vi "fruitWay.vi"() -> ()   [LabVIEW 2014]
uses:
  <vilib>/Utility/file.llb/Write To Spreadsheet File (DBL).vi
panel:
  out "appended array":dbl[][](array[numeric])
  out "Array 2":dbl[](array[numeric])
  out "Array":dbl[](array[numeric])
  in  "Boolean":bool
  in  "initial angle":dbl
  in  "initial velocity":dbl
  in  "Position:Top":i32
  in  "Position:Left":i32
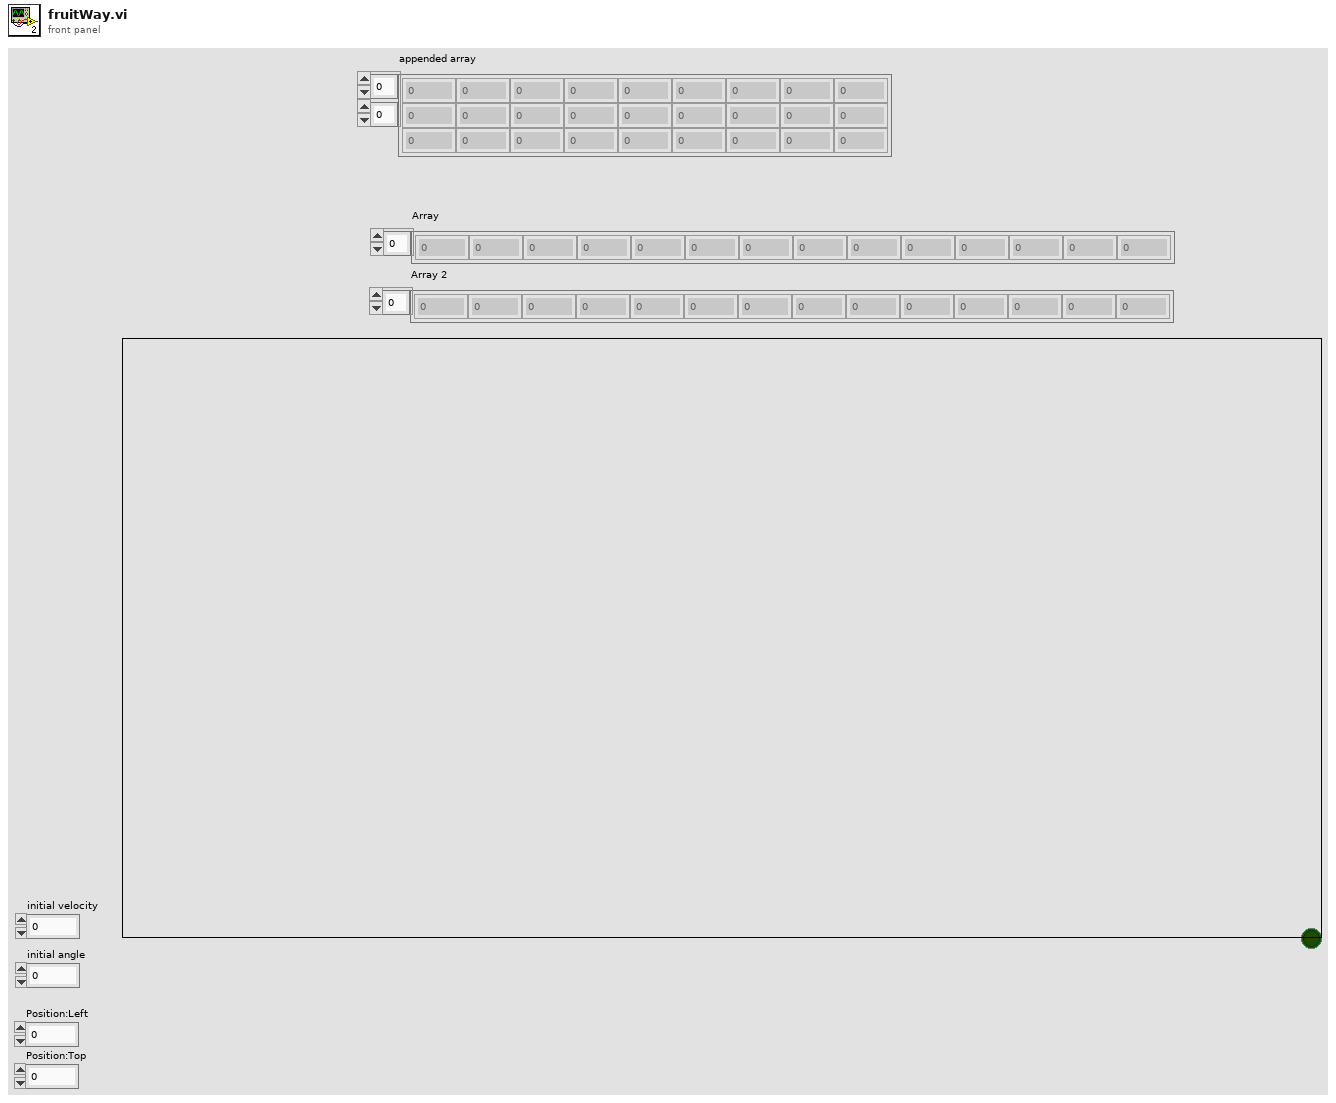
[diagram p1: front panel]
types:
  T1 = typedef "LVPositionTypeDef.ctl" = cluster{"Left":i32, "Top":i32}
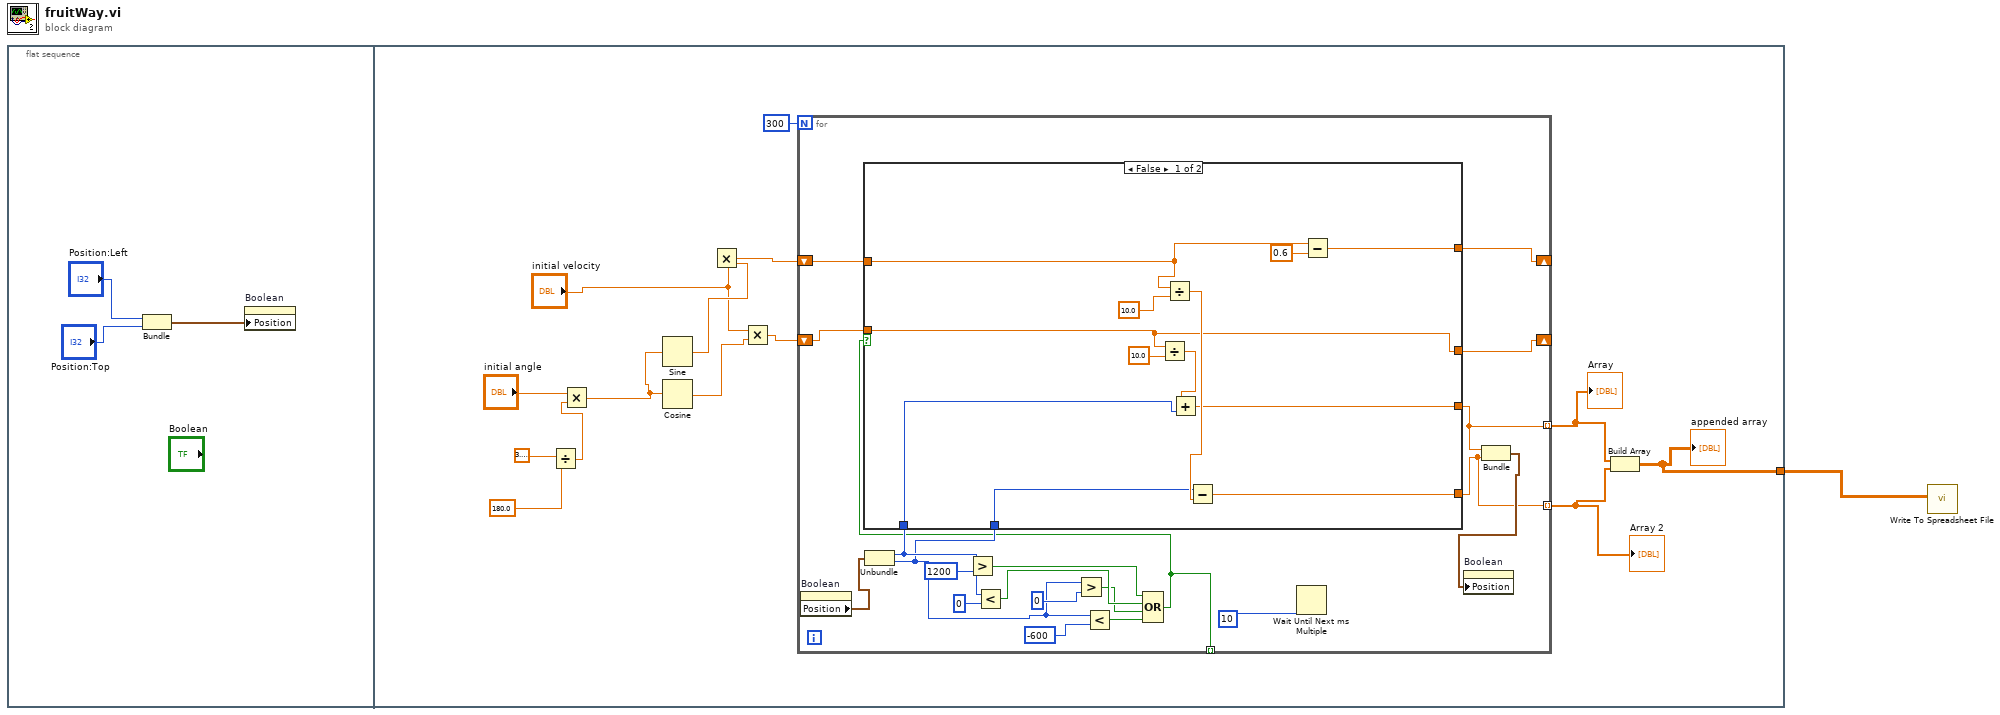
[diagram p0: block diagram]
diagram:
  n1 = flat-sequence {
    tunnel: [w5] -> w1
    frame #0 {
      n2 = Bundle("Position:Left"="Position:Left", "Position:Top"="Position:Top") -> (w2:cluster{"Position:Left":i32, "Position:Top":i32})  [unwired: 1 in]
      n3 = property on="Boolean" class="Bool (strict)"("Position"=w2) -> ()  [unwired: 2 in, 2 out]
    }
    frame #1 {
      n4 = Divide(x=3.141592653589793, y=180.0) -> (x/y=w13:dbl)
      n5 = Multiply(x="initial angle", y=w13) -> (x*y=w11:dbl)
      n6 = Sine(x=w11) -> (sin(x)=w18:dbl)
      n7 = Cosine(x=w11) -> (cos(x)=w16:dbl)
      n8 = Multiply(x="initial velocity", y=w18) -> (x*y=w10:dbl)
      n9 = Multiply(x="initial velocity", y=w16) -> (x*y=w9:dbl)
      n10 = for {
        N: 300 -> [_]
        shift-right: [w27] -> _
        shift-left: w10 -> [w30]
        shift-right: [w28] -> _
        shift-left: w9 -> [w29]
        tunnel: [w24] -> w6 mode=indexing
        tunnel: [w20] -> _ mode=indexing
        tunnel: [w19] -> w7 mode=indexing
        n11 = property on="Boolean" class="Bool (strict)"() -> ("Position"=w22:T1)  [unwired: 2 in, 2 out]
        n12 = Unbundle(w22) -> ("Left"=w26:i32, "Top"=w25:i32)
        n13 = Greater?(x=w26, y=1200) -> (0:w34:bool)
        n14 = Less?(x=w26, y=0) -> (x < y?=w33:bool)
        n15 = Greater?(x=w25, y=0) -> (0:w32:bool)
        n16 = Less?(x=w25, y=-600) -> (x < y?=w31:bool)
        n17 = Compound Arithmetic op=OR(w34, w33, w32, w31) -> (w20:bool)
        n18 = case shown="False" w20 {
          tunnel: w30 -> [w47 w53]
          tunnel: w29 -> [w39 w54]
          tunnel: [w39 w54] -> w28
          tunnel: [w46 w53] -> w27
          tunnel: w26 -> [w44 w52]
          tunnel: w25 -> [w43 w51]
          tunnel: [w42 w52] -> w24
          tunnel: [w41 w51] -> w19
          frame False {
            n19 = Divide(x=w39, y=10.0) -> (x/y=w40:dbl)
            n20 = Divide(x=w47, y=10.0) -> (x/y=w45:dbl)
            n21 = Add(x=w40, y=w44) -> (x+y=w42:dbl)
            n22 = Subtract(x=w43, y=w45) -> (x-y=w41:dbl)
            n23 = Subtract(x=w47, y=0.6) -> (x-y=w46:dbl)
          }
          frame True {
          }
        }
        n24 = Wait Until Next ms Multiple(millisecond multiple=u32 10) -> ()  [unwired: 1 out]
        n25 = Bundle("Left"=w24, "Top"=w19) -> (w21:cluster{"Left":dbl, "Top":dbl})  [unwired: 1 in]
        n26 = property on="Boolean" class="Bool (strict)"("Position"=w21) -> ()  [unwired: 2 in, 2 out]
      }
      "Array" <- w6
      "Array 2" <- w7
      n27 = Build Array(w6, w7) -> (w5:dbl[][])
      "appended array" <- w5
    }
  }
  n28 = call-poly <vilib>:"Write To Spreadsheet File.vi"("2D data"=w1) -> ()  [unwired: 7 in, 1 out]
